vi "digitally_ros_final.vi"() -> ()   [LabVIEW 2019]
uses:
  <vilib>/addons/eal4LabVIEW/eal4LabVIEW.lvlib
  <vilib>/addons/eal4LabVIEW/ApiLib/Connection control/ealApiConnect_string.vi
panel:
  out "Is the PID finished?":bool
  out "Iteration counter loop 1":i32
  out "Init success\\fail":i32
  out "Deviation 3":dbl
  out "Deviation 2":dbl
  out "Deviation 1":dbl
  out "Sensor values":dbl[](array[numeric])
  out "List length":i32
  in  "Loop 3":bool
  in  "Loop 2":bool
  out "Iteration counter loop 3":i32
  out "In Range? (1)":bool
  out "In Range? (2)":bool
  out "In Range? (3)":bool
  in  "condition 6":i32(ring) items=["AXIS_CONDITION_ACTIVE"=0, "AXIS_CONDITION_PARKING"=1, "AXIS_CONDITION_DEACTIVATED"=2, "AXIS_CONDITION_ACTIVE_DECOUPLED"=4, "AXIS_CONDITION_PARKING_DECOUPLED"=5, "AXIS_CONDITION_DEACTIVATED_DECOUPLED"=6, "AXIS_CONDITION_ACTIVE_PARAMETERIZATION"=8, "AXIS_CONDITION_PARKING_PARAMETERIZATION"=9, "AXIS_CONDITION_DEACTIVATED_PARAMETERIZATION"=10, "AXIS_CONDITION_ACTIVE_DECOUPLED_PARAMETERIZATION"=12, "AXIS_CONDITION_PARKING_DECOUPLED_PARAMETERIZATION"=13, "AXIS_CONDITION_DEACTIVATED_DECOUPLED_PARAMETERIZATION"=14]
  in  "slave index 6":i32
  in  "condition 5":i32(ring) items=["AXIS_CONDITION_ACTIVE"=0, "AXIS_CONDITION_PARKING"=1, "AXIS_CONDITION_DEACTIVATED"=2, "AXIS_CONDITION_ACTIVE_DECOUPLED"=4, "AXIS_CONDITION_PARKING_DECOUPLED"=5, "AXIS_CONDITION_DEACTIVATED_DECOUPLED"=6, "AXIS_CONDITION_ACTIVE_PARAMETERIZATION"=8, "AXIS_CONDITION_PARKING_PARAMETERIZATION"=9, "AXIS_CONDITION_DEACTIVATED_PARAMETERIZATION"=10, "AXIS_CONDITION_ACTIVE_DECOUPLED_PARAMETERIZATION"=12, "AXIS_CONDITION_PARKING_DECOUPLED_PARAMETERIZATION"=13, "AXIS_CONDITION_DEACTIVATED_DECOUPLED_PARAMETERIZATION"=14]
  in  "slave index 5":i32
  in  "condition 4":i32(ring) items=["AXIS_CONDITION_ACTIVE"=0, "AXIS_CONDITION_PARKING"=1, "AXIS_CONDITION_DEACTIVATED"=2, "AXIS_CONDITION_ACTIVE_DECOUPLED"=4, "AXIS_CONDITION_PARKING_DECOUPLED"=5, "AXIS_CONDITION_DEACTIVATED_DECOUPLED"=6, "AXIS_CONDITION_ACTIVE_PARAMETERIZATION"=8, "AXIS_CONDITION_PARKING_PARAMETERIZATION"=9, "AXIS_CONDITION_DEACTIVATED_PARAMETERIZATION"=10, "AXIS_CONDITION_ACTIVE_DECOUPLED_PARAMETERIZATION"=12, "AXIS_CONDITION_PARKING_DECOUPLED_PARAMETERIZATION"=13, "AXIS_CONDITION_DEACTIVATED_DECOUPLED_PARAMETERIZATION"=14]
  in  "slave index 4":i32
  out "RPM Boom":dbl
  out "RPM Arm":dbl
  out "RPM Bucket":dbl
  in  "Loop 1":bool
  out "Return value lab_2.py":dbl[](array[numeric])
  out "Iteration counter loop 2":i32
  # "PID Control"
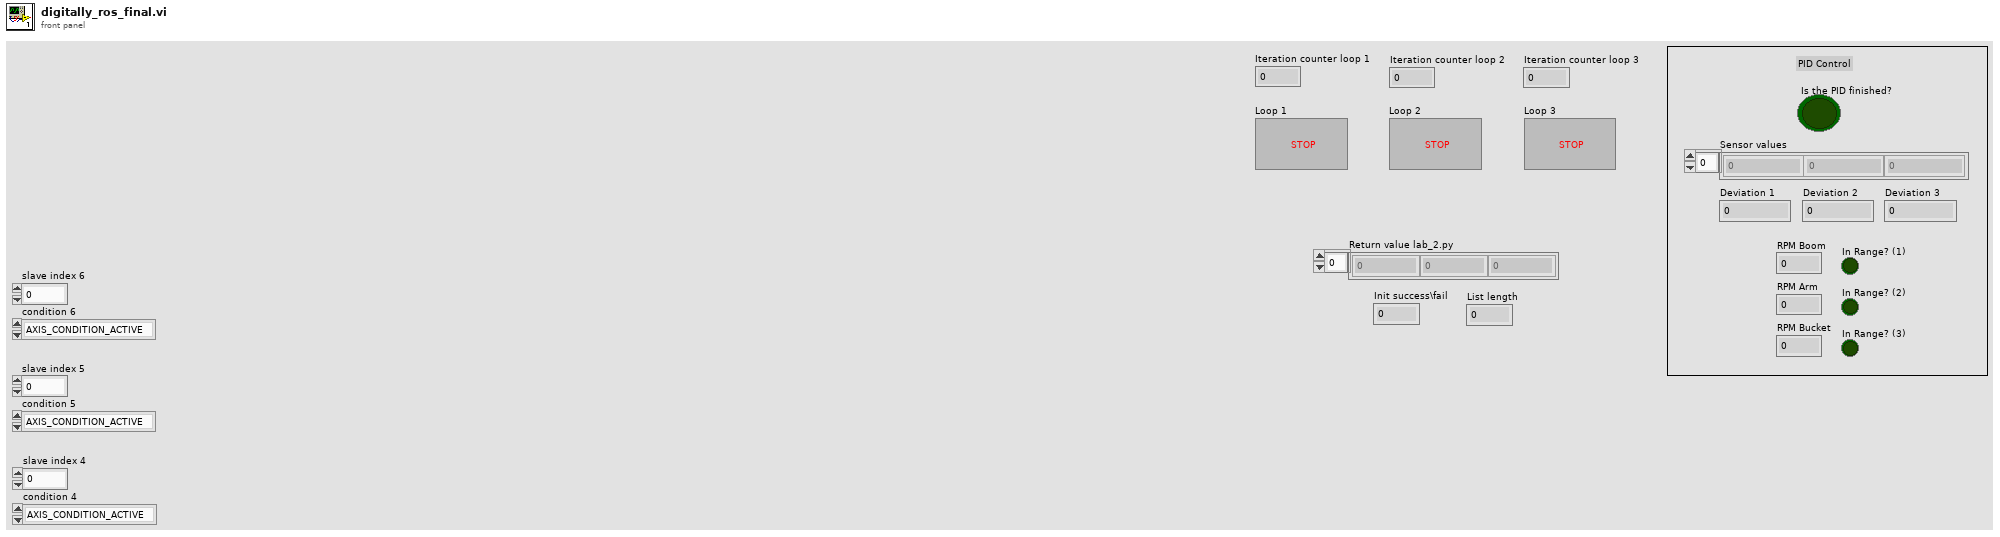
[diagram p1: front panel]
types:
  T1 = cluster{"Velocity":dbl, "Acceleration":dbl, "Deceleration":dbl, "Jerk":dbl}
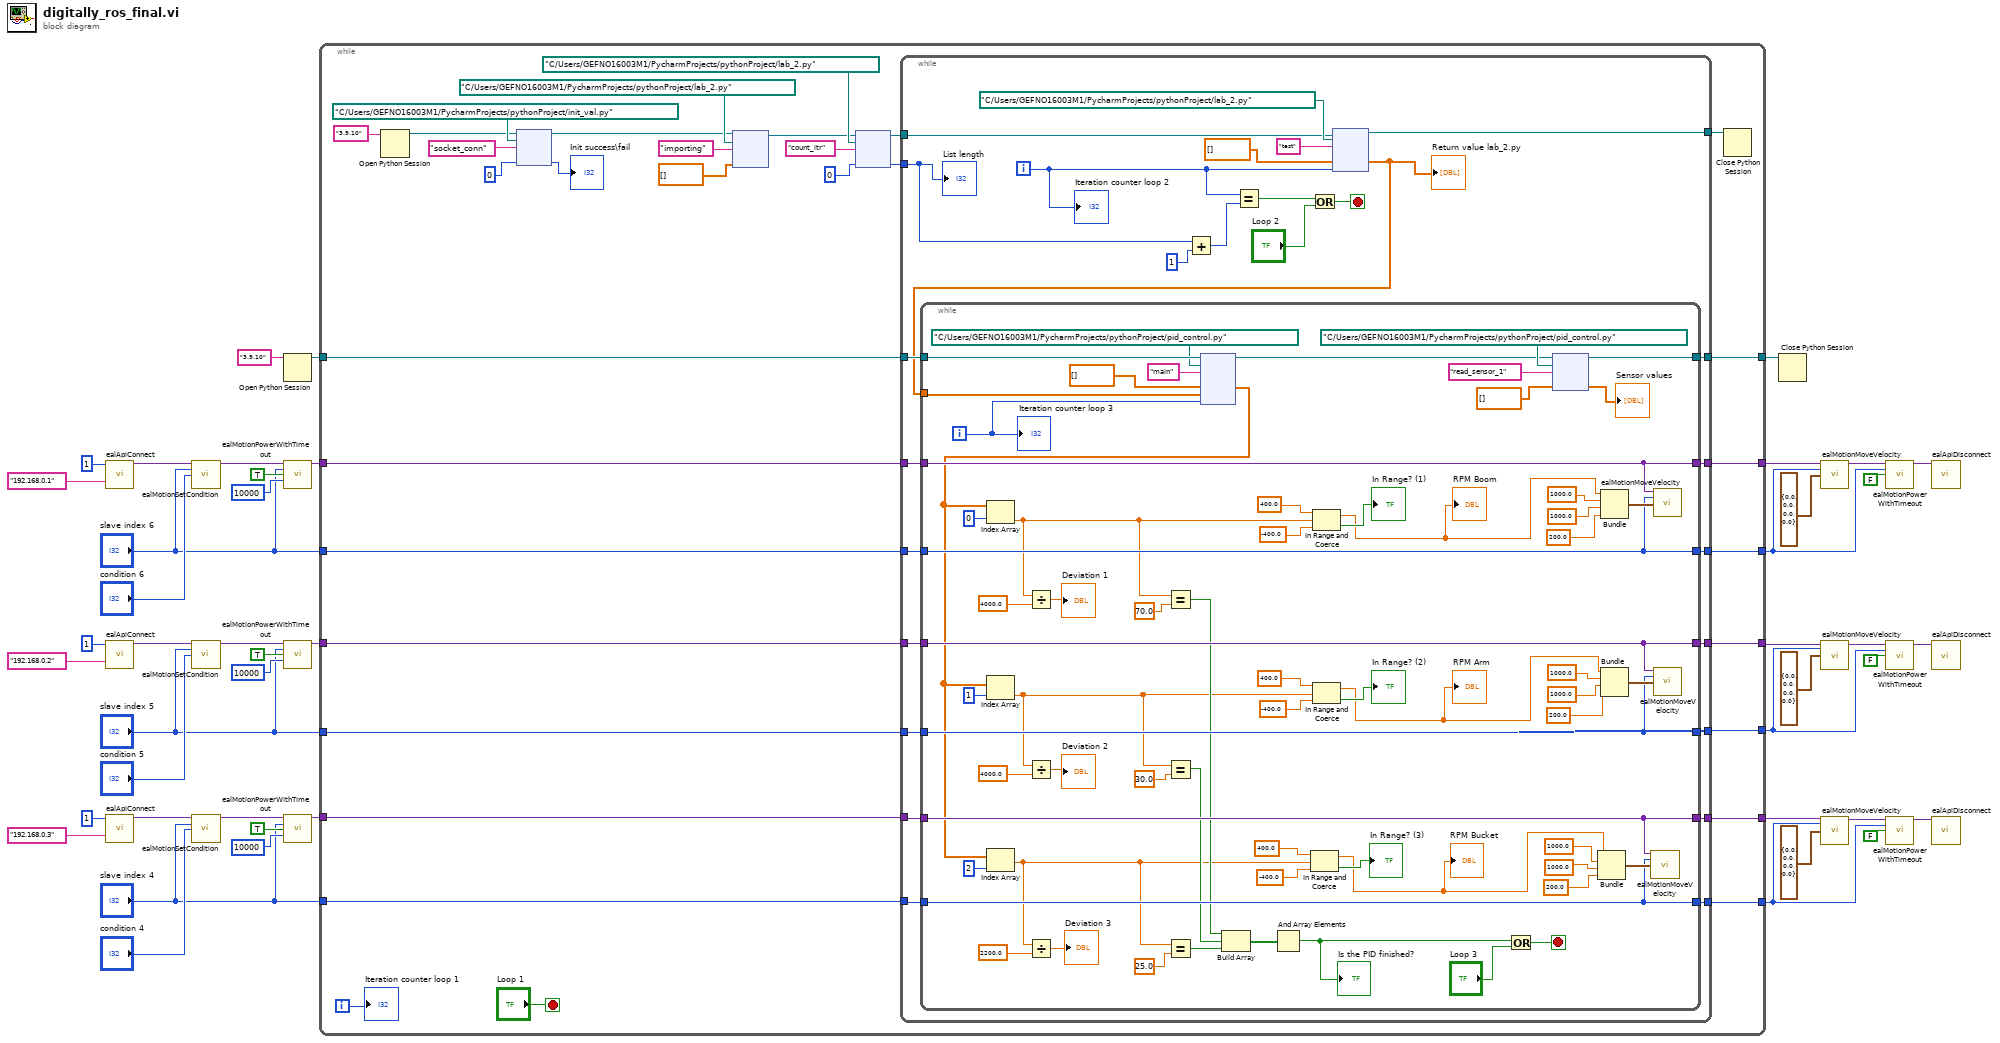
[diagram p0: block diagram]
diagram:
  n1 = call-poly <vilib>:"ealApiConnect.vi"("maximum no of axes"=1, "ip address"="192.168.0.1") -> ("connection out"=w20:variant)  [unwired: 12 in, 1 out]
  n2 = call-poly <vilib>:"ealApiConnect.vi"("maximum no of axes"=1, "ip address"="192.168.0.2") -> ("connection out"=w27:variant)  [unwired: 12 in, 1 out]
  n3 = call-poly <vilib>:"ealApiConnect.vi"("maximum no of axes"=1, "ip address"="192.168.0.3") -> ("connection out"=w34:variant)  [unwired: 12 in, 1 out]
  n4 = call <vilib>:"ealMotionSetCondition.vi"("connection in"=w20, "slave index"="slave index 6", "condition"="condition 6") -> ("connection out"=w19:variant)  [unwired: 11 in, 1 out]
  n5 = call <vilib>:"ealMotionSetCondition.vi"("connection in"=w27, "slave index"="slave index 5", "condition"="condition 5") -> ("connection out"=w26:variant)  [unwired: 11 in, 1 out]
  n6 = call <vilib>:"ealMotionSetCondition.vi"("connection in"=w34, "slave index"="slave index 4", "condition"="condition 4") -> ("connection out"=w33:variant)  [unwired: 11 in, 1 out]
  n7 = Open Python Session(python version="3.9.10" ("Python version")) -> (session out=w5:refnum<k35>)  [unwired: 2 in, 1 out]
  n8 = call <vilib>:"ealMotionPowerWithTimeout.vi"("connection in"=w19, "slave index"="slave index 6", "value"=TRUE, "timeout"=10000) -> ("connection out"=w15:variant)  [unwired: 10 in, 1 out]
  n9 = call <vilib>:"ealMotionPowerWithTimeout.vi"("connection in"=w26, "slave index"="slave index 5", "value"=TRUE, "timeout"=10000) -> ("connection out"=w14:variant)  [unwired: 10 in, 1 out]
  n10 = call <vilib>:"ealMotionPowerWithTimeout.vi"("connection in"=w33, "slave index"="slave index 4", "value"=TRUE, "timeout"=10000) -> ("connection out"=w13:variant)  [unwired: 10 in, 1 out]
  n11 = while {
    tunnel: w15 -> [w80]
    tunnel: w14 -> [w79]
    tunnel: w13 -> [w78]
    tunnel: [w67] -> w12
    tunnel: [w77] -> w1
    tunnel: "slave index 6" -> [w76]
    tunnel: "slave index 5" -> [w75]
    tunnel: [w74] -> w9
    tunnel: [w70] -> w8
    tunnel: "slave index 4" -> [w73]
    tunnel: w5 -> [w72]
    tunnel: [w68] -> w4
    tunnel: [w71] -> w3
    tunnel: [w69] -> w2
    i -> [w53]
    stop <- "Loop 1" stop-if-true
    n12 = Open Python Session(python version="3.9.10" ("Python version")) -> (session out=w51:refnum<k35>)  [unwired: 2 in, 1 out]
    n13 = node(w51, path "C:/Users/GEFNO16003M1/PycharmProjects/pythonProject/init_val.py" ("module path"), "socket_conn" ("function name"), 0) -> (w55:refnum<k35>, →"Init success\\fail":i32)  [unwired: 1 in, 3 out]
    n14 = node(w55, path "C:/Users/GEFNO16003M1/PycharmProjects/pythonProject/lab_2.py" ("module path"), "importing" ("function name"), dbl[] []) -> (w61:refnum<k35>)  [unwired: 2 in, 3 out]
    n15 = node(w61, path "C:/Users/GEFNO16003M1/PycharmProjects/pythonProject/lab_2.py" ("module path"), "count_itr" ("function name"), 0) -> (w60:refnum<k35>, w58:i32)  [unwired: 1 in, 3 out]
    n16 = while {
      tunnel: [w104] -> w50
      tunnel: w60 -> [w106]
      tunnel: w58 -> [w84]
      tunnel: w80 -> [w103]
      tunnel: w79 -> [w93]
      tunnel: w78 -> [w102]
      tunnel: [w95] -> w67
      tunnel: [w96] -> w77
      tunnel: w76 -> [w94]
      tunnel: w75 -> [w92]
      tunnel: [w97] -> w74
      tunnel: w73 -> [w99]
      tunnel: w72 -> [w91]
      tunnel: [w101] -> w68
      tunnel: [w100] -> w71
      tunnel: [w98] -> w70
      tunnel: [w90] -> w69
      i -> [w83]
      stop <- w89 stop-if-true
      n17 = Add(x=w84, y=1) -> (x+y=w86:i32)
      n18 = Equal?(x=w83, y=w86) -> (x = y?=w87:bool)
      n19 = Or(x=w87, y="Loop 2") -> (x .or. y?=w89:bool)
      n20 = node(w106, path "C:/Users/GEFNO16003M1/PycharmProjects/pythonProject/lab_2.py" ("module path"), "test" ("function name"), dbl[] [], w83) -> (w104:refnum<k35>, w82:dbl[])  [unwired: 2 in, 3 out]
      "Return value lab_2.py" <- w82
      n21 = while {
        tunnel: w82 -> [w127]
        tunnel: w103 -> [w145]
        tunnel: w102 -> [w147]
        tunnel: [w147] -> w101
        tunnel: [w146] -> w100
        tunnel: w99 -> [w146]
        tunnel: [w143] -> w98
        tunnel: [w142] -> w97
        tunnel: [w144] -> w96
        tunnel: [w145] -> w95
        tunnel: w94 -> [w144]
        tunnel: w93 -> [w143]
        tunnel: w92 -> [w142]
        tunnel: w91 -> [w141]
        tunnel: [w126] -> w90
        i -> [w113]
        stop <- w129 stop-if-true
        n22 = node(w141, path "C:/Users/GEFNO16003M1/PycharmProjects/pythonProject/pid_control.py" ("module path"), "main" ("function name"), dbl[] [], w127, w113) -> (w121:refnum<k35>, w140:dbl[])  [unwired: 3 in, 3 out]
        n23 = Index Array(array=w140, index=0) -> (element=w111:dbl)
        n24 = Index Array(array=w140, index=1) -> (element=w110:dbl)
        n25 = Index Array(array=w140, index=2) -> (element=w109:dbl)
        n26 = Divide(x=w111, y=4000.0) -> (x/y=→"Deviation 1":dbl)
        n27 = Divide(x=w110, y=4000.0) -> (x/y=→"Deviation 2":dbl)
        n28 = Divide(x=w109, y=2200.0) -> (x/y=→"Deviation 3":dbl)
        n29 = Equal?(x=w111, y=70.0) -> (x = y?=w136:bool)
        n30 = Equal?(x=w110, y=30.0) -> (x = y?=w135:bool)
        n31 = Equal?(x=w109, y=25.0) -> (x = y?=w134:bool)
        n32 = Build Array(w136, w135, w134) -> (w133:bool[])
        n33 = And Array Elements(Boolean array=w133) -> (logical AND=w114:bool)
        "Is the PID finished?" <- w114
        n34 = In Range and Coerce(upper limit=400.0, x=w109, lower limit=-400.0) -> (coerced(x)=w130:dbl, In Range?=→"In Range? (3)":bool)
        "RPM Bucket" <- w130
        n35 = In Range and Coerce(upper limit=400.0, x=w111, lower limit=-400.0) -> (coerced(x)=w132:dbl, In Range?=→"In Range? (1)":bool)
        "RPM Boom" <- w132
        n36 = In Range and Coerce(upper limit=400.0, x=w110, lower limit=-400.0) -> (coerced(x)=w131:dbl, In Range?=→"In Range? (2)":bool)
        "RPM Arm" <- w131
        n37 = Or(x=w114, y="Loop 3") -> (x .or. y?=w129:bool)
        n38 = node(w121, path "C:/Users/GEFNO16003M1/PycharmProjects/pythonProject/pid_control.py" ("module path"), "read_sensor_1" ("function name"), dbl[] []) -> (w126:refnum<k35>, →"Sensor values":dbl[])  [unwired: 1 in, 3 out]
        n39 = Bundle("upper limit"=w130, 1000.0, 1000.0, 200.0) -> (w167:cluster{"upper limit":dbl, dbl, dbl, dbl})  [unwired: 1 in]
        n40 = Bundle("upper limit"=w132, 1000.0, 1000.0, 200.0) -> (w157:cluster{"upper limit":dbl, dbl, dbl, dbl})  [unwired: 1 in]
        n41 = Bundle("upper limit"=w131, 1000.0, 1000.0, 200.0) -> (w162:cluster{"upper limit":dbl, dbl, dbl, dbl})  [unwired: 1 in]
        n42 = call <vilib>:"ealMotionMoveVelocity.vi"("connection in"=w147, "slave index"=w146, "parameters set"=w167) -> ()  [unwired: 11 in, 2 out]
        n43 = call <vilib>:"ealMotionMoveVelocity.vi"("connection in"=w145, "slave index"=w144, "parameters set"=w157) -> ()  [unwired: 11 in, 2 out]
        n44 = call <vilib>:"ealMotionMoveVelocity.vi"("connection in"=w143, "slave index"=w142, "parameters set"=w162) -> ()  [unwired: 11 in, 2 out]
        "Iteration counter loop 3" <- w113
      }
      "Iteration counter loop 2" <- w83
      "List length" <- w84
    }
    n45 = Close Python Session(session in=w50) -> ()  [unwired: 1 in, 1 out]
    "Iteration counter loop 1" <- w53
  }
  n46 = Close Python Session(session in=w2) -> ()  [unwired: 1 in, 1 out]
  n47 = call <vilib>:"ealMotionMoveVelocity.vi"("connection in"=w12, "slave index"=w1, "parameters set"=T1 {"Velocity"=0.0, "Acceleration"=0.0, "Deceleration"=0.0, "Jerk"=0.0}) -> ("connection out"=w39:variant)  [unwired: 11 in, 1 out]
  n48 = call <vilib>:"ealMotionMoveVelocity.vi"("connection in"=w8, "slave index"=w9, "parameters set"=T1 {"Velocity"=0.0, "Acceleration"=0.0, "Deceleration"=0.0, "Jerk"=0.0}) -> ("connection out"=w43:variant)  [unwired: 11 in, 1 out]
  n49 = call <vilib>:"ealMotionMoveVelocity.vi"("connection in"=w4, "slave index"=w3, "parameters set"=T1 {"Velocity"=0.0, "Acceleration"=0.0, "Deceleration"=0.0, "Jerk"=0.0}) -> ("connection out"=w47:variant)  [unwired: 11 in, 1 out]
  n50 = call <vilib>:"ealMotionPowerWithTimeout.vi"("connection in"=w39, "slave index"=w1, "value"=FALSE) -> ("connection out"=w40:variant)  [unwired: 11 in, 1 out]
  n51 = call <vilib>:"ealMotionPowerWithTimeout.vi"("connection in"=w43, "slave index"=w9, "value"=FALSE) -> ("connection out"=w44:variant)  [unwired: 11 in, 1 out]
  n52 = call <vilib>:"ealMotionPowerWithTimeout.vi"("connection in"=w47, "slave index"=w3, "value"=FALSE) -> ("connection out"=w48:variant)  [unwired: 11 in, 1 out]
  n53 = call <vilib>:"ealApiDisconnect.vi"("connection in"=w40) -> ()  [unwired: 14 in, 1 out]
  n54 = call <vilib>:"ealApiDisconnect.vi"("connection in"=w44) -> ()  [unwired: 14 in, 1 out]
  n55 = call <vilib>:"ealApiDisconnect.vi"("connection in"=w48) -> ()  [unwired: 14 in, 1 out]
